vi "Load Settings from XML - Copy.vi"(8 "error in (no error)":errorcluster, 11 "Settings in":T1={"Hardware Configuration"={"DAQmx Channel"="cDAQETH/ai0:23, cDAQETH/ai29, cDAQETH/ai31:30", "Sample Rate"=1000.0, "DAQmx Task"="", "ResetInterp"=FALSE, "GainConstants"=[0.01, 2.0, 10.0, 1.0, 0.1], "Simulate"=FALSE, "FilterCoefficients"=[[1.0], [1.0]], "ChannelNames"=["CH1X", "CH1Y", "CH1Z", "CH2X", "CH2Y", "CH2Z", "CH3X", "CH3Y", "CH3Z", "CH4X", "CH4Y", "CH4Z", "CH5X", "CH5Y", "CH5Z", "CH6X", "CH6Y", "CH6Z", "CH7X", "CH7Y", "CH7Z", "CH8X", "CH8Y", "CH8Z"], "ActiveChannels"=[], "Display Rate"=0, "ResponseExtension"=TRUE}, "Logging Configuration"={"Log File Base Path"=path "D:/Documents/LabVIEW Data/Logged Data.tdms", "Samples to Save"=9900, "Trigger - Threshold"=0.0, "Trigger - Channel"=0, "Always Log"=FALSE, "External Trigger"=TRUE, "External Trigger Armed"=FALSE, "TDMS File Reference"=refnum, "DAQVersion"="1.0", "SWVersion"="1.7.5.12", "CircSamples"=100, "BeepWhenComplete"=TRUE, "ChannelConfig"=[["CH1", "CH1", "NA", "XYZ"], ["CH2", "CH2", "NA", "XYZ"], ["CH3", "CH3", "NA", "XYZ"], ["CH4", "CH4", "NA", "XYZ"], ["CH5", "CH5", "NA", "XYZ"], ["CH6", "CH6", "NA", "XYZ"], ["CH7", "CH7", "NA", "XYZ"], ["CH8", "CH8", "NA", "XYZ"]], "ActiveChannels"=[], "Title"="Title", "Description"="Description....", "ChannelNames"=["CH1X", "CH1Y", "CH1Z", "CH2X", "CH2Y", "CH2Z", "CH3X", "CH3Y", "CH3Z", "CH4X", "CH4Y", "CH4Z", "CH5X", "CH5Y", "CH5Z", "CH6X", "CH6Y", "CH6Z", "CH7X", "CH7Y", "CH7Z", "CH8X", "CH8Y", "CH8Z"], "ResponseExtension"=TRUE}}) -> (0 "error out":errorcluster, 3 "Settings out":T1={"Hardware Configuration"={"DAQmx Channel"="", "Sample Rate"=0.0, "DAQmx Task"="", "ResetInterp"=FALSE, "GainConstants"=[], "Simulate"=FALSE, "FilterCoefficients"=[], "ChannelNames"=[], "ActiveChannels"=[], "Display Rate"=1000, "ResponseExtension"=TRUE}, "Logging Configuration"={"Log File Base Path"=path "", "Samples to Save"=0, "Trigger - Threshold"=0.0, "Trigger - Channel"=0, "Always Log"=FALSE, "External Trigger"=FALSE, "External Trigger Armed"=FALSE, "TDMS File Reference"=refnum, "DAQVersion"="", "SWVersion"="", "CircSamples"=0, "BeepWhenComplete"=FALSE, "ChannelConfig"=[], "ActiveChannels"=[], "Title"="", "Description"="", "ChannelNames"=[], "ResponseExtension"=TRUE}})   [LabVIEW 2017, in "Settings.lvlib"]
doc: "Attempts to load previous user specified settings from an XML file.\n\nThis VI will not generate an error. If a suitable XML file can't be loaded and parsed then it will simply return the default settings."
uses:
  Settings.lvlib
  Settings.ctl
  Acquisition/Hardware Configuration.ctl
  Logging/Logging Configuration.ctl
  <vilib>/Utility/file.llb/Read Delimited Spreadsheet (DBL).vi
  <vilib>/Utility/xml.llb/Read From XML File(string).vi
  <vilib>/Utility/xml.llb/Write to XML File(string).vi
  <resource>/objmgr/daqmx.rc
  Acquisition/Acquisition.lvlib
  Logging/Logging.lvlib
panel:
  # "(Scroll up for Settings Controls)"
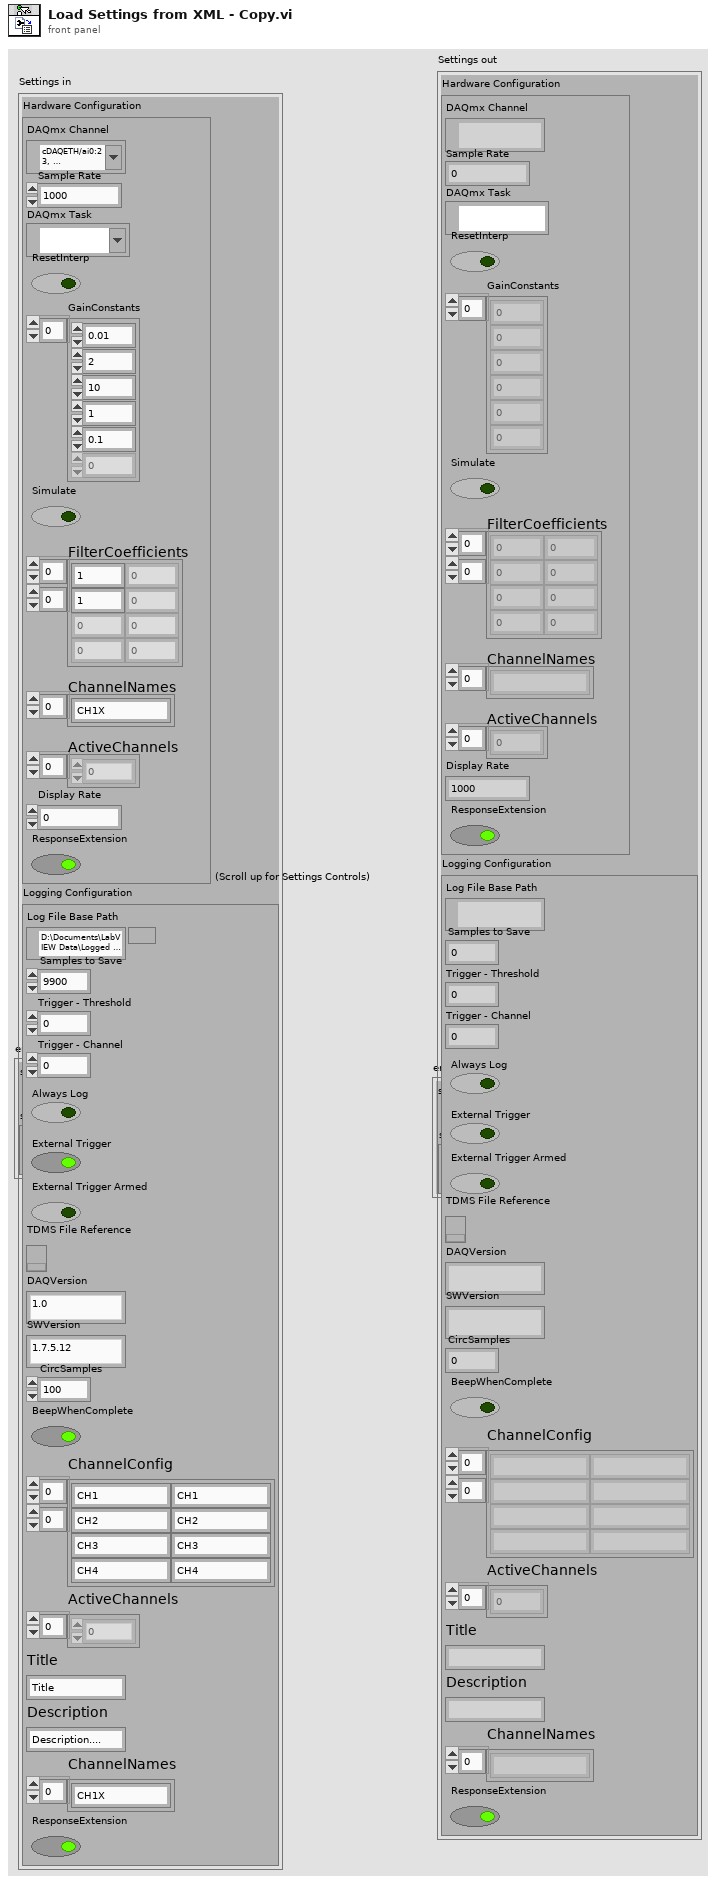
[diagram p1: front panel]
types:
  T1 = typedef "Settings.lvlib/Settings.ctl" = cluster{"Hardware Configuration":T2, "Logging Configuration":T3}
  T2 = typedef "Acquisition.lvlib/Hardware Configuration.ctl" = cluster{"DAQmx Channel":tag, "Sample Rate":dbl, "DAQmx Task":refnum<k21>, "ResetInterp":bool, "GainConstants":dbl[], "Simulate":bool, "FilterCoefficients":dbl[][], "ChannelNames":string[], "ActiveChannels":i32[], "Display Rate":i32, "ResponseExtension":bool}
  T3 = typedef "Logging.lvlib/Logging Configuration.ctl" = cluster{"Log File Base Path":path, "Samples to Save":u32, "Trigger - Threshold":dbl, "Trigger - Channel":u32, "Always Log":bool, "External Trigger":bool, "External Trigger Armed":bool, "TDMS File Reference":refnum<k34>, "DAQVersion":string, "SWVersion":string, "CircSamples":u32, "BeepWhenComplete":bool, "ChannelConfig":string[][], "ActiveChannels":i32[], "Title":string, "Description":string, "ChannelNames":string[], "ResponseExtension":bool}
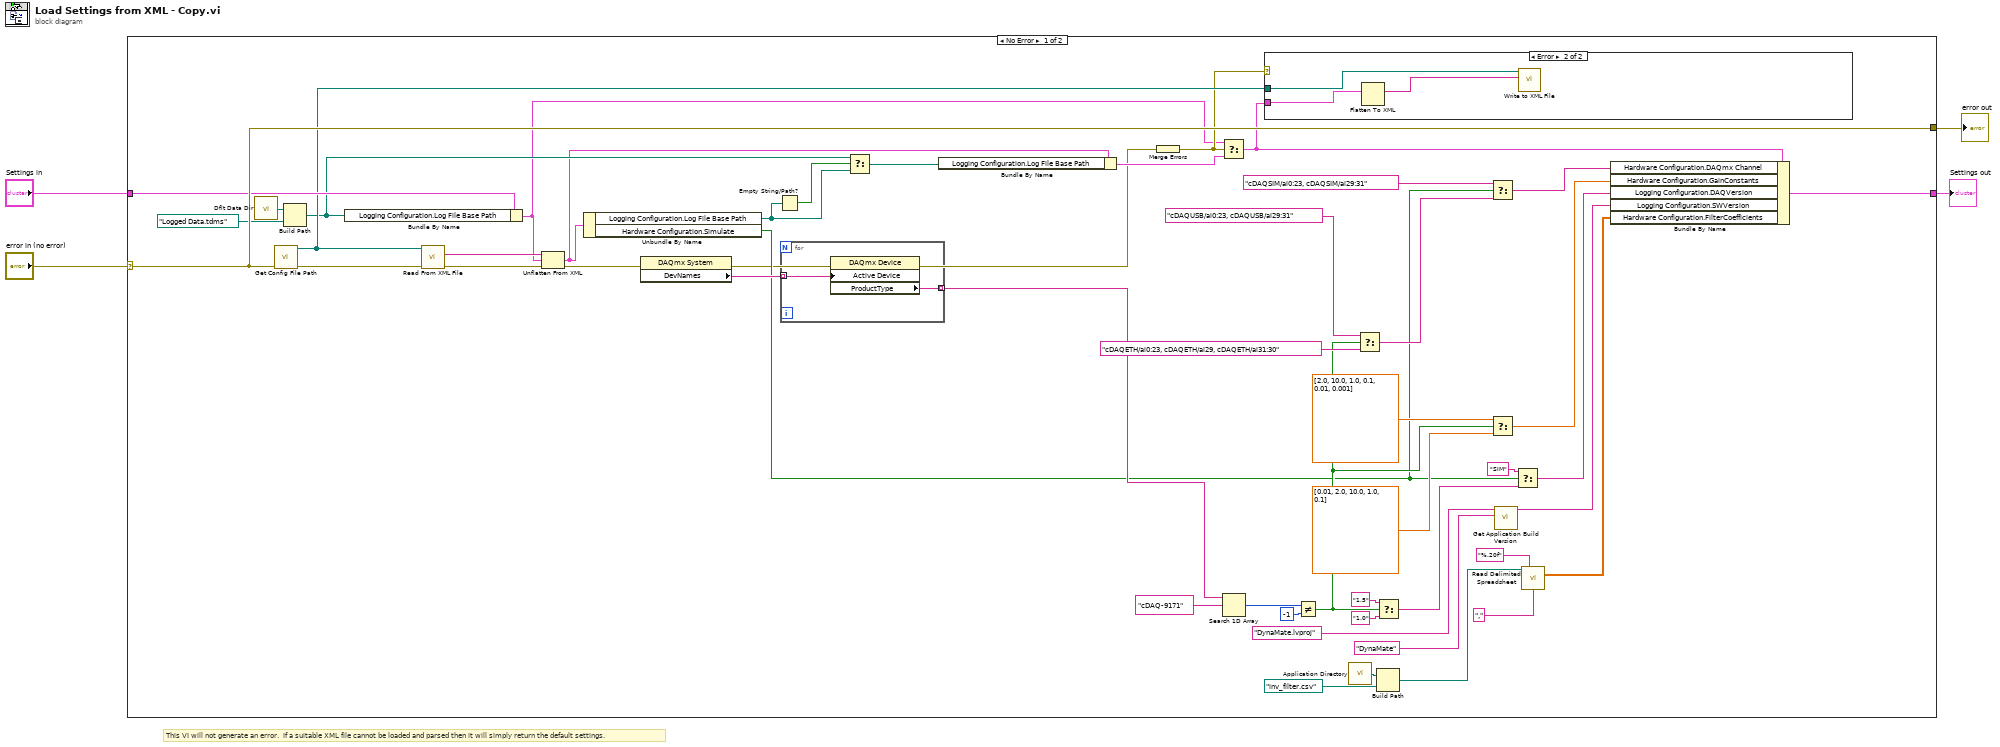
[diagram p0: block diagram]
diagram:
  # "This VI will not generate an error.  If a suitable XML file cannot be loaded and parsed then it will simply return the default settings."
  n1 = case shown="No Error" "error in (no error)" {
    selector: "error in (no error)" -> [w51 w60]
    tunnel: [w51 w60] -> w3
    tunnel: "Settings in" -> [w50 w59]
    tunnel: [w36 w59] -> w1
    frame No Error {
      n2 = call <vilib>:"Dflt Data Dir.vi"() -> ("App:Default Data Directory"=w49:path)
      n3 = call "Get Config File Path.vi"("error in (no error)"=w51) -> ("error out"=w53:errorcluster, "XML File Path"=w47:path)  [unwired: 9 in]
      n4 = Build Path(base path=w49, name or relative path=path "Logged Data.tdms" ("App:Default Data Directory")) -> (appended path=w41:path)
      n5 = Bundle By Name(cluster=w50, "Logging Configuration.Log File Base Path"=w41) -> (w6:T1)
      n6 = call-poly <vilib>:"Read From XML File.vi"("error in (no error)"=w53, "XML File Path"=w47) -> ("error out"=w46:errorcluster, "XML Elements"=w52:string)  [unwired: 7 in, 1 out]
      n7 = Unflatten From XML(xml string=w52, type=w6, error in (no error)=w46) -> (value=w37:T1, error out=w38:errorcluster)
      n8 = Unbundle By Name(w37) -> ("Logging Configuration.Log File Base Path"=w42:path, "Hardware Configuration.Simulate"=w14:bool)
      n9 = property class="DAQmx System"(error in=w38) -> (error out=w5:errorcluster, "DevNames"=w39:tag[])  [unwired: 1 in, 1 out]
      n10 = Empty String/Path?(string/path=w42) -> (empty?=w45:bool)
      n11 = for {
        tunnel: w39 -> [w54] mode=indexing
        tunnel: [w55] -> w34 mode=indexing
        n12 = property class="DAQmx Device"("Active Device"=w54) -> ("ProductType"=w55:string)  [unwired: 2 in, 2 out]
      }
      n13 = Select(t=w41, s=w45, f=w42) -> (s? t:f=w44:path)
      n14 = Bundle By Name(cluster=w37, "Logging Configuration.Log File Base Path"=w44) -> (w43:T1)
      n15 = Merge Errors(w5) -> (w40:errorcluster)
      n16 = Select(t=w6, s=w40, f=w43) -> (s? t:f=w35:T1)
      n17 = Search 1D Array(1D array=w34, element="cDAQ-9171") -> (index of element=w32:i32)  [unwired: 1 in]
      n18 = case shown="Error" w40 {
        tunnel: w35 -> [_ w58]
        tunnel: w47 -> [_ w56]
        frame No Error {
        }
        frame Error {
          n19 = Flatten To XML(anything=w58) -> (xml string=w57:string)
          n20 = call-poly <vilib>:"Write to XML File.vi"("XML Input"=w57, "XML File Path"=w56) -> ()  [unwired: 7 in, 3 out]
        }
      }
      n21 = Not Equal?(x=w32, y=-1) -> (x != y?=w24:bool)
      n22 = call <vilib>:"Application Directory.vi"() -> ("Application Directory"=w8:path)
      n23 = Select(t=tag "cDAQUSB/ai0:23, cDAQUSB/ai29:31" ("Hardware Configuration.DAQmx Channel"), s=w24, f=tag "cDAQETH/ai0:23, cDAQETH/ai29, cDAQETH/ai31:30" ("Hardware Configuration.DAQmx Channel")) -> (s? t:f=w18:tag)
      n24 = Build Path(base path=w8, name or relative path=path "inv_filter.csv" ("file path (dialog if empty)")) -> (appended path=w7:path)
      n25 = Select(t="1.5", s=w24, f="1.0") -> (s? t:f=w17:string)
      n26 = Select(t=tag "cDAQSIM/ai0:23, cDAQSIM/ai29:31" ("Hardware Configuration.DAQmx Channel"), s=w14, f=w18) -> (s? t:f=w13:tag)
      n27 = Select(t=dbl[] [2.0, 10.0, 1.0, 0.1, 0.01, 0.001], s=w24, f=dbl[] [0.01, 2.0, 10.0, 1.0, 0.1]) -> (s? t:f=w27:dbl[])
      n28 = call "Get Application Build Version.vi"("Build Specification Name"="DynaMate", "Project Filename"="DynaMate.lvproj") -> ("Version String"=w21:string)  [unwired: 7 in, 2 out]
      n29 = Select(t="SIM", s=w14, f=w17) -> (s? t:f=w15:string)
      n30 = call-poly <vilib>:"Read Delimited Spreadsheet.vi"("file path (dialog if empty)"=w7, "format (%.3f)"="%.20f", "delimiter (\\t)"="," ("delimiter (\\t)")) -> ("all rows"=w10:dbl[][])  [unwired: 7 in, 5 out]
      n31 = Bundle By Name(cluster=w35, "Hardware Configuration.DAQmx Channel"=w13, "Hardware Configuration.GainConstants"=w27, "Logging Configuration.DAQVersion"=w15, "Logging Configuration.SWVersion"=w21, "Hardware Configuration.FilterCoefficients"=w10) -> (w36:T1)
    }
    frame Error {
    }
  }
  "error out" <- w3
  "Settings out" <- w1
